vi "Extract Array Variable.vi"(1 "In array":dbl[](array[numeric]), 2 "Cluster Key":u16) -> (0 "Out Variable":dbl)   [LabVIEW 2020]
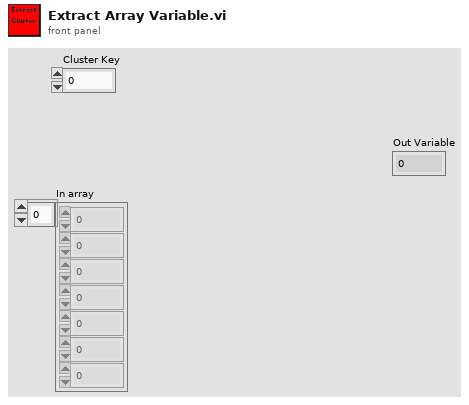
[diagram p1: front panel]
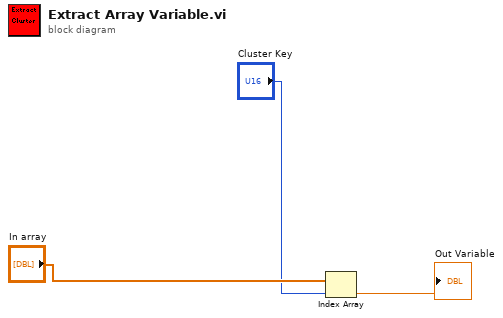
[diagram p0: block diagram]
diagram:
  n1 = Index Array(array="In array", index="Cluster Key") -> (element=→"Out Variable":dbl)
